vi "Demo3-Display_Trace.vi"() -> ()   [LabVIEW 2020]
panel:
  out "Diode Trace":waveform(dbl)[](graph)
  out "Live Responses":string[](array[string])
  out "Device Keywords":string[](array[string])
  in  "IP Address of Remote Device":string="196.254.31.200"
  in  "Disconnect":bool
  # "Diode Demo - Display ADC Trace"
  # "Demonstrates display of the ADC trace, with background and signal regions masked, for the STM32 Diode Device."
  # "VI Instructions\n\n1. Make sure you know the Device IP Address.\n2. From Windows command prompt, confirm ping to IP address.\n3. Type the correct device IP address into this VI.\n3. Run this VI. *Note:* Only one TCP connection to the device's SCPI-like server can run at a time.\n4. When finished, disconnect safely from the device via the \"Disconnect\" toggle button. (Not the Abort button).\n\nCreated by Scott Feister on July 13, 2022."
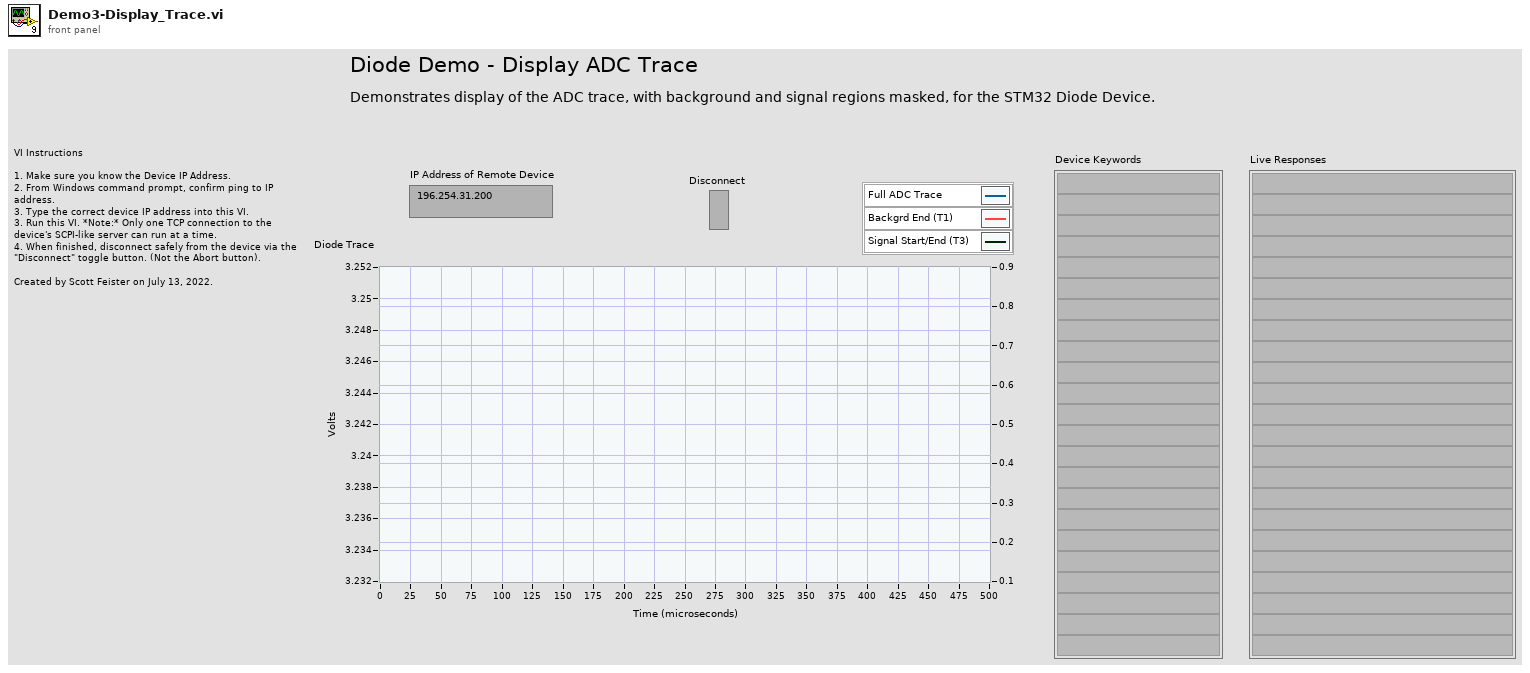
[diagram p1: front panel]
types:
  T1 = typedef "DDAQ-Keyword.ctl" = cluster{"Keyword":string, "Gettable":bool, "Settable":bool, "Is Array":bool, "Data Type":string, "Description":string}
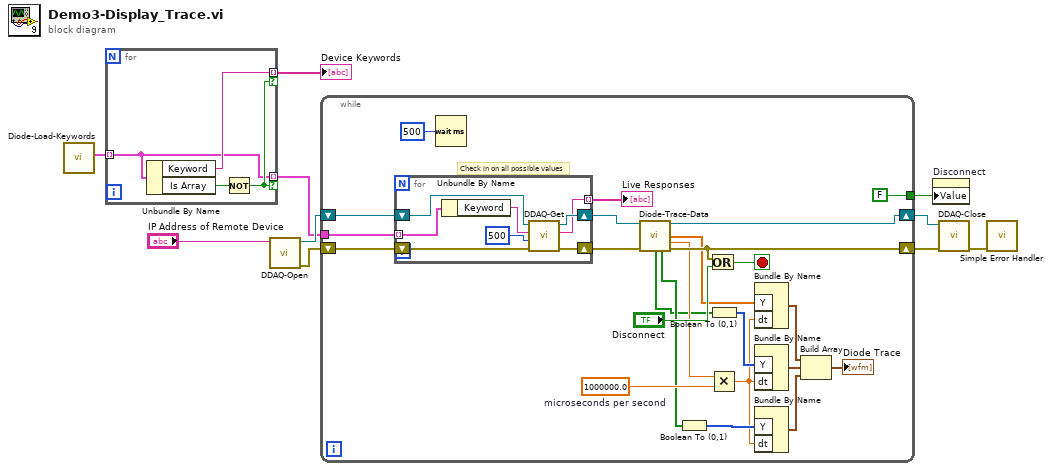
[diagram p0: block diagram]
diagram:
  n1 = call "Diode-Load-Keywords.vi"() -> ("Diodes Keywords Array"=w3:T1[])  [unwired: 11 in]
  n2 = for {
    tunnel: w3 -> [w11] mode=indexing
    tunnel: [w14] -> w2 mode=indexing if=w12
    tunnel: [w11] -> w1 mode=indexing if=w12
    n3 = Unbundle By Name(w11) -> ("Keyword"=w14:string, "Is Array"=w13:bool)
    n4 = Not(x=w13) -> (.not. x?=w12:bool)
  }
  "Device Keywords" <- w2
  n5 = call "DDAQ-Open.vi"("IP Address of Nucleo Device"="IP Address of Remote Device") -> ("error out"=w9:errorcluster, "connection ID"=w10:refnum<k5>)  [unwired: 8 in, 1 out]
  n6 = while {
    shift-right: [w27] -> w8
    shift-left: w10 -> [w38]
    shift-right: [w28] -> w7
    shift-left: w9 -> [w37]
    tunnel: [FALSE] -> w5
    tunnel: w1 -> [w31]
    stop <- w33 stop-if-true
    w24 = 1000000.0  # microseconds per second
    # "Check in on all possible values"
    n7 = for {
      shift-right: [w44] -> w30
      shift-left: w38 -> [w46]
      shift-right: [w43] -> w29
      shift-left: w37 -> [w45]
      tunnel: [w41] -> w32 mode=indexing
      tunnel: w31 -> [w40] mode=indexing
      n8 = Unbundle By Name(w40) -> ("Keyword"=w39:string)
      n9 = call "DDAQ-Get.vi"("error in (no error)"=w45, "max bytes to read (10000)"=500 ("max bytes to read (500)"), "SCPI-like Keyword (leave off question mark)"=w39, "connection ID"=w46) -> ("error out"=w43:errorcluster, "Response"=w41:string, "connection ID out"=w44:refnum<k5>)  [unwired: 3 in, 2 out]
    }
    "Live Responses" <- w32
    n10 = Wait (ms)(milliseconds to wait=u32 500) -> ()  [unwired: 1 out]
    n11 = call "Diode-Trace-Data.vi"("connection ID"=w30, "error in (no error)"=w29) -> ("connection ID out"=w27:refnum<k5>, "Trace (Volts)"=w26:dbl[], "dt"=w25:dbl, "Background Mask Array"=w15:bool[], "Signal Mask Array"=w16:bool[], "error out"=w28:errorcluster)  [unwired: 5 in, 3 out]
    n12 = Boolean To (0,1)(Boolean=w16) -> (0, 1=w22:i16[])
    n13 = Or(x=w28, y="Disconnect") -> (x .or. y?=w33:bool)
    n14 = Boolean To (0,1)(Boolean=w15) -> (0, 1=w23:i16[])
    n15 = Multiply(x=w25, y=w24) -> (x*y=w21:dbl)
    n16 = Bundle By Name("Y"=w26, "dt"=w21) -> (w18:waveform(dbl))  [unwired: 1 in]
    n17 = Bundle By Name("Y"=w23, "dt"=w21) -> (w20:waveform(i16))  [unwired: 1 in]
    n18 = Bundle By Name("Y"=w22, "dt"=w21) -> (w19:waveform(i16))  [unwired: 1 in]
    n19 = Build Array(w18, w20, w19) -> (→"Diode Trace":waveform(dbl)[])
  }
  n20 = property on="Disconnect" class="Bool (strict)"("Value"=w5) -> ()  [unwired: 2 in, 2 out]
  n21 = call "DDAQ-Close.vi"("error in (no error)"=w7, "connection ID"=w8) -> ("error out"=w6:errorcluster)  [unwired: 8 in, 1 out]
  n22 = call <vilib>:"Simple Error Handler.vi"("error in (no error)"=w6) -> ()  [unwired: 4 in, 5 out]
